vi "Timing Functions.vi"() -> ()   [LabVIEW 2015]
panel:
  in  "Stop":bool
  out "Green":bool
  out "Amber":bool
  out "Red":bool
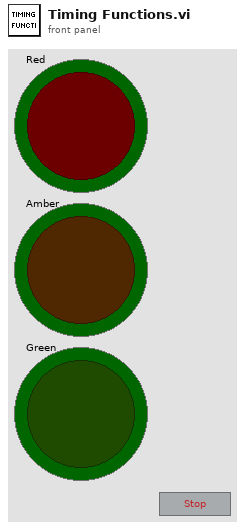
[diagram p1: front panel]
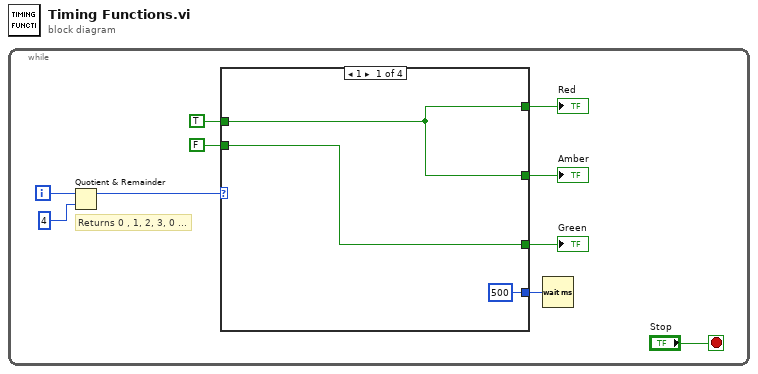
[diagram p0: block diagram]
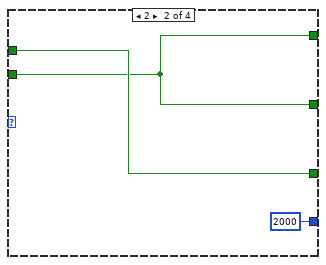
[diagram p2: hidden frame]
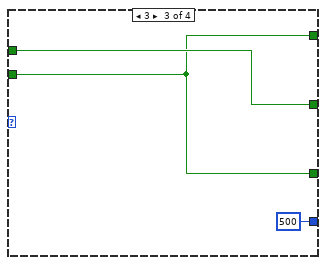
[diagram p3: hidden frame]
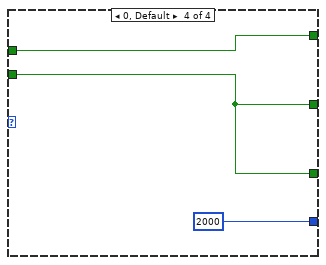
[diagram p4: hidden frame]
diagram:
  n1 = while {
    i -> [w10]
    stop <- "Stop" stop-if-true
    # "Returns 0 , 1, 2, 3, 0 ..."
    n2 = Quotient & Remainder(x=w10, y=4) -> (x-y*floor(x/y)=w8:i32)  [unwired: 1 out]
    n3 = case shown="1" w8 {
      tunnel: [w13 w15 w18 w22] -> w7
      tunnel: [w13 w15 w19 w21] -> w6
      tunnel: [w12 w16 w18 w21] -> w5
      tunnel: TRUE -> [w13 w16 w19 w22]
      tunnel: FALSE -> [w12 w15 w18 w21]
      tunnel: [u32 500 ("milliseconds to wait") u32 2000 ("milliseconds to wait") u32 500 ("milliseconds to wait") u32 2000 ("milliseconds to wait")] -> w2
      frame 1 {
      }
      frame 2 {
      }
      frame 3 {
      }
      frame 0, Default {
      }
    }
    "Amber" <- w6
    "Green" <- w5
    "Red" <- w7
    n4 = Wait (ms)(milliseconds to wait=w2) -> ()  [unwired: 1 out]
  }
